vi "DSOX2014A pilot sample subVI.vi"(8 "error in (no error)":errorcluster, 11 "VISA Refnum in":refnum<visa-resource-name>) -> (0 "error out":errorcluster, 2 "Array":dbl[](array[numeric]), 3 "VISA Refnum out":refnum<visa-resource-name>)   [LabVIEW 2016]
uses:
  <instrlib>/Agilent 2000 3000 X-Series/Public/Data/Read Measurement (Current Value).vi
  <instrlib>/Agilent 2000 3000 X-Series/Agilent 2000 3000 X-Series.lvlib
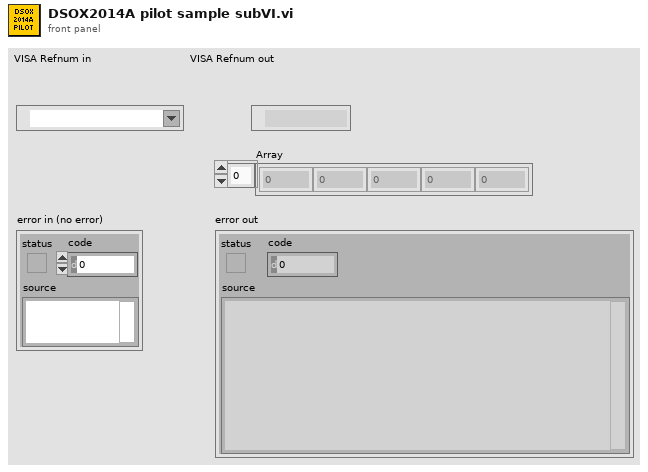
[diagram p1: front panel]
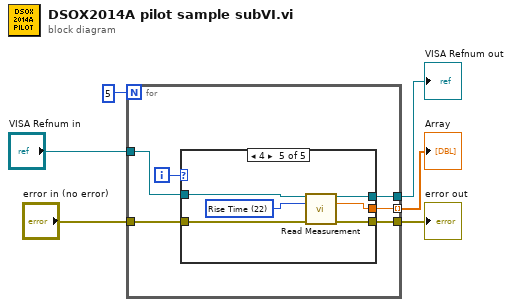
[diagram p0: block diagram]
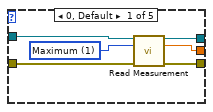
[diagram p2: hidden frame]
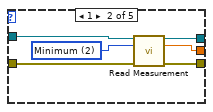
[diagram p3: hidden frame]
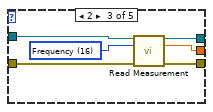
[diagram p4: hidden frame]
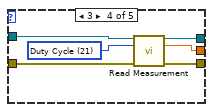
[diagram p5: hidden frame]
diagram:
  n1 = for {
    N: 5 -> [_]
    tunnel: "error in (no error)" -> [w11]
    tunnel: [w10] -> w3
    tunnel: "VISA Refnum in" -> [w9]
    tunnel: [w8] -> w4
    tunnel: [w7] -> w5 mode=indexing
    i -> [w12]
    n2 = case shown="4" w12 {
      tunnel: w11 -> [w16 w22 w25 w32 w40]
      tunnel: [w13 w21 w26 w33 w38] -> w10
      tunnel: w9 -> [w17 w24 w29 w36 w41]
      tunnel: [w18 w23 w28 w35 w42] -> w8
      tunnel: [w14 w19 w27 w34 w37] -> w7
      frame 0, Default {
        w15 = 1 items=["Peak-Peak", "Maximum", "Minimum", "Amplitude", "Top", "Base", "Overshoot", "Preshoot", "Average - N Cycles", "Average - Full Screen", "DC RMS - N Cycles", "DC RMS - Full Screen", "AC RMS - N Cycles", "AC RMS - Full Screen (Std Dev)", "Ratio", "Period", "Frequency", "Counter", "+Width", "-Width", "Burst Width", "Duty Cycle", "Rise Time", "Fall Time", "Delay", "Phase", "X minY", "X maxY", "Positive Pulse Count", "Negative Pulse Count", "Raising Edge Count", "Falling Edge Count", "Area - N Cycle", "Area - Full Screen", "Nth Edge Time", "Nth Edge Cross Level Time"] ("Measurement Type (0: Peak-Peak) 3")
        n3 = call-poly <instrlib>:"Read Measurement.vi"("VISA resource name"=w17, "Measurement Type (0: Peak-Peak)"=w15, "error in (no error)"=w16) -> ("VISA resource name out"=w18:refnum<visa-resource-name>, "Result Value"=w14:dbl, "error out"=w13:errorcluster)  [unwired: 10 in]
      }
      frame 1 {
        w20 = 2 items=["Peak-Peak", "Maximum", "Minimum", "Amplitude", "Top", "Base", "Overshoot", "Preshoot", "Average - N Cycles", "Average - Full Screen", "DC RMS - N Cycles", "DC RMS - Full Screen", "AC RMS - N Cycles", "AC RMS - Full Screen (Std Dev)", "Ratio", "Period", "Frequency", "Counter", "+Width", "-Width", "Burst Width", "Duty Cycle", "Rise Time", "Fall Time", "Delay", "Phase", "X minY", "X maxY", "Positive Pulse Count", "Negative Pulse Count", "Raising Edge Count", "Falling Edge Count", "Area - N Cycle", "Area - Full Screen", "Nth Edge Time", "Nth Edge Cross Level Time"] ("Measurement Type (0: Peak-Peak)")
        n4 = call-poly <instrlib>:"Read Measurement.vi"("VISA resource name"=w24, "Measurement Type (0: Peak-Peak)"=w20, "error in (no error)"=w22) -> ("VISA resource name out"=w23:refnum<visa-resource-name>, "Result Value"=w19:dbl, "error out"=w21:errorcluster)  [unwired: 10 in]
      }
      frame 2 {
        w30 = 16 items=["Peak-Peak", "Maximum", "Minimum", "Amplitude", "Top", "Base", "Overshoot", "Preshoot", "Average - N Cycles", "Average - Full Screen", "DC RMS - N Cycles", "DC RMS - Full Screen", "AC RMS - N Cycles", "AC RMS - Full Screen (Std Dev)", "Ratio", "Period", "Frequency", "Counter", "+Width", "-Width", "Burst Width", "Duty Cycle", "Rise Time", "Fall Time", "Delay", "Phase", "X minY", "X maxY", "Positive Pulse Count", "Negative Pulse Count", "Raising Edge Count", "Falling Edge Count", "Area - N Cycle", "Area - Full Screen", "Nth Edge Time", "Nth Edge Cross Level Time"] ("Measurement Type (0: Peak-Peak) 2")
        n5 = call-poly <instrlib>:"Read Measurement.vi"("VISA resource name"=w29, "Measurement Type (0: Peak-Peak)"=w30, "error in (no error)"=w25) -> ("VISA resource name out"=w28:refnum<visa-resource-name>, "Result Value"=w27:dbl, "error out"=w26:errorcluster)  [unwired: 10 in]
      }
      frame 3 {
        w31 = 21 items=["Peak-Peak", "Maximum", "Minimum", "Amplitude", "Top", "Base", "Overshoot", "Preshoot", "Average - N Cycles", "Average - Full Screen", "DC RMS - N Cycles", "DC RMS - Full Screen", "AC RMS - N Cycles", "AC RMS - Full Screen (Std Dev)", "Ratio", "Period", "Frequency", "Counter", "+Width", "-Width", "Burst Width", "Duty Cycle", "Rise Time", "Fall Time", "Delay", "Phase", "X minY", "X maxY", "Positive Pulse Count", "Negative Pulse Count", "Raising Edge Count", "Falling Edge Count", "Area - N Cycle", "Area - Full Screen", "Nth Edge Time", "Nth Edge Cross Level Time"] ("Measurement Type (0: Peak-Peak) 2")
        n6 = call-poly <instrlib>:"Read Measurement.vi"("VISA resource name"=w36, "Measurement Type (0: Peak-Peak)"=w31, "error in (no error)"=w32) -> ("VISA resource name out"=w35:refnum<visa-resource-name>, "Result Value"=w34:dbl, "error out"=w33:errorcluster)  [unwired: 10 in]
      }
      frame 4 {
        w39 = 22 items=["Peak-Peak", "Maximum", "Minimum", "Amplitude", "Top", "Base", "Overshoot", "Preshoot", "Average - N Cycles", "Average - Full Screen", "DC RMS - N Cycles", "DC RMS - Full Screen", "AC RMS - N Cycles", "AC RMS - Full Screen (Std Dev)", "Ratio", "Period", "Frequency", "Counter", "+Width", "-Width", "Burst Width", "Duty Cycle", "Rise Time", "Fall Time", "Delay", "Phase", "X minY", "X maxY", "Positive Pulse Count", "Negative Pulse Count", "Raising Edge Count", "Falling Edge Count", "Area - N Cycle", "Area - Full Screen", "Nth Edge Time", "Nth Edge Cross Level Time"] ("Measurement Type (0: Peak-Peak) 2")
        n7 = call-poly <instrlib>:"Read Measurement.vi"("VISA resource name"=w41, "Measurement Type (0: Peak-Peak)"=w39, "error in (no error)"=w40) -> ("VISA resource name out"=w42:refnum<visa-resource-name>, "Result Value"=w37:dbl, "error out"=w38:errorcluster)  [unwired: 10 in]
      }
    }
  }
  "error out" <- w3
  "VISA Refnum out" <- w4
  "Array" <- w5
